vi "tmdl_resp.vi"(8 "error in (no error)":errorcluster, 9 "DL Rx Timeout (ms)":u32, 10 "Active Dut":T1, 11 "Refnum in":refnum<k20>) -> (0 "error out":errorcluster, 3 "Boolean":bool, 5 "Received Text":string)   [LabVIEW 2018]
uses:
  Resources_Test/UART/ControlTestSlot.ctl
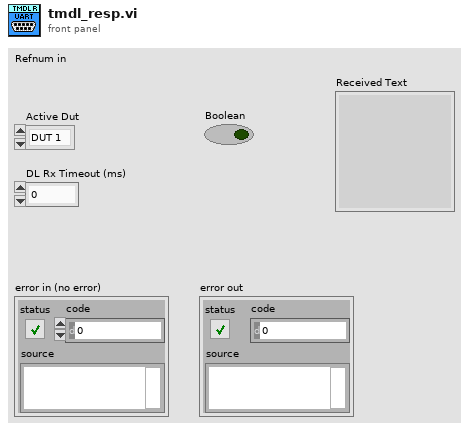
[diagram p1: front panel]
types:
  T1 = typedef "ControlTestSlot.ctl" = enum16{"DUT 1", "DUT 2"}
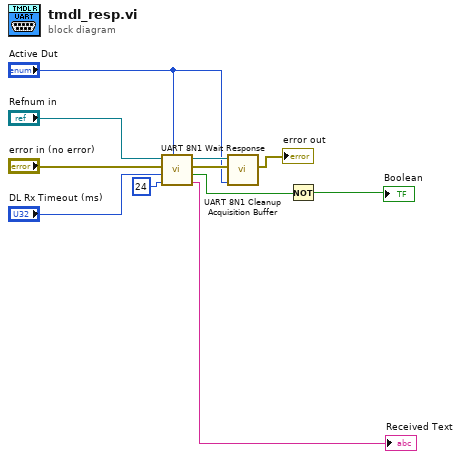
[diagram p0: block diagram]
diagram:
  n1 = call "UART 8N1 Wait Response.vi"("Active Dut"="Active Dut", "Response Size (char)"=u32 24, "Response Timeout (ms)"="DL Rx Timeout (ms)", "Error In"="error in (no error)", "FPGA VI Reference In"="Refnum in") -> ("Received Text"=→"Received Text":string, "Timeout Flag"=w5:bool, "Error Out"=w3:errorcluster, "FPGA VI Reference Out"=w4:refnum<k20>)  [unwired: 2 in, 1 out]
  n2 = call "UART 8N1 Cleanup Acquisition Buffer.vi"("Active Dut"="Active Dut", "Error In"=w3, "FPGA VI Reference In"=w4) -> ("Error Out"=→"error out":errorcluster)  [unwired: 6 in, 2 out]
  n3 = Not(x=w5) -> (.not. x?=→"Boolean":bool)
